vi "Error monitor FVG.vi"(6 "length (10)":i32=10, 7 "Akcja (SET)":T1=enum."SET", 8 "error in (no error)":errorcluster, 9 "acq czas":dbl=0.01953125) -> (0 "error out":errorcluster, 1 "Czasy Array":dbl[](array[numeric]), 2 "Error Array":errorcluster[](array[cluster]))   [LabVIEW 2013]
doc: "Use this template to build a VI to use as a subVI."
uses:
  Kontrolki/FVGs/FVG akcje podstawowa.ctl
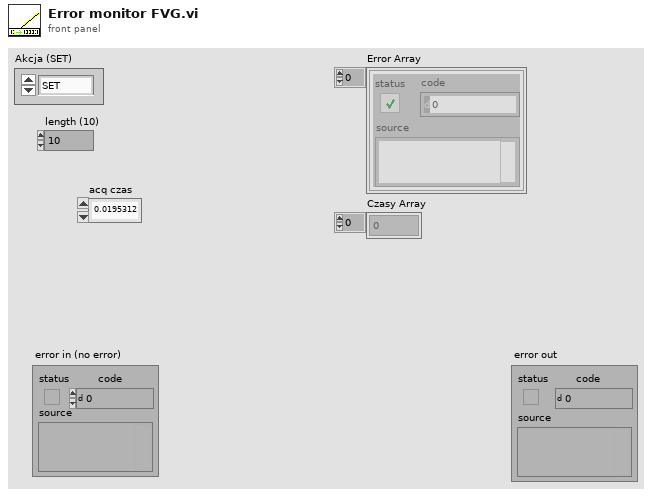
[diagram p1: front panel]
types:
  T1 = typedef "FVG akcje podstawowa.ctl" = enum16{"GET", "SET"}
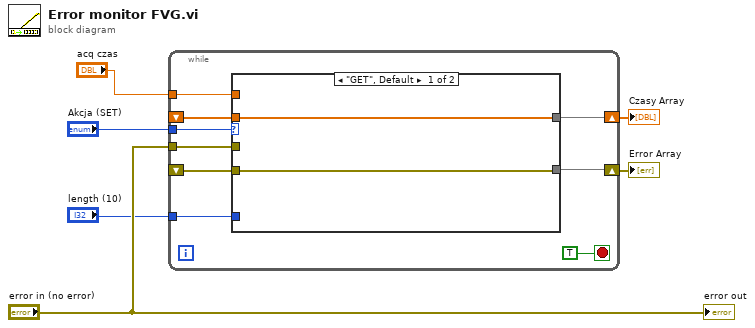
[diagram p0: block diagram]
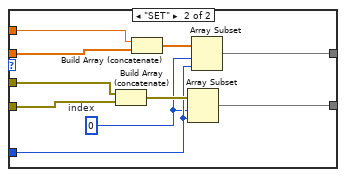
[diagram p2: hidden frame]
diagram:
  n1 = while {
    tunnel: "error in (no error)" -> [w14]
    tunnel: "Akcja (SET)" -> [w13]
    shift-right: [w12] -> w4
    shift-left: _ -> [w11]
    tunnel: "length (10)" -> [w10]
    tunnel: "acq czas" -> [w9]
    shift-right: [w8] -> w1
    shift-left: _ -> [w7]
    stop <- TRUE stop-if-true
    n2 = case shown="\"GET\", Default" w13 {
      tunnel: w14 -> [_ w27]
      tunnel: [w17 w24] -> w12
      tunnel: w11 -> [w17 w26]
      tunnel: w10 -> [_ w19]
      tunnel: w9 -> [_ w22]
      tunnel: [w16 w21] -> w8
      tunnel: w7 -> [w16 w20]
      frame "GET", Default {
      }
      frame "SET" {
        w18 = 0  # index
        n3 = Build Array (concatenate)(w27, w26) -> (w25:errorcluster[])
        n4 = Build Array (concatenate)(w22, w20) -> (w23:dbl[])
        n5 = Array Subset(array=w25, index=w18, length=w19) -> (w24:errorcluster[])
        n6 = Array Subset(array=w23, index=w18, length=w19) -> (w21:dbl[])
      }
    }
  }
  "Error Array" <- w4
  "Czasy Array" <- w1
  "error out" <- "error in (no error)"
